vi "Complex Dot Product.vi"(2 "Y Vector":cdb[](array[numeric]) format="%.2f", 3 "X Vector":cdb[](array[numeric]) format="%.2f") -> (0 "error":i32, 1 "X * Y":cdb format="%.2f")   [LabVIEW 2017, in "NI_AALBase.lvlib"]
doc: "Computes the dot product of <B>X Vector</B> and <B>Y Vector</B>. The data types you wire to the <B>X Vector</B> and <B>Y Vector</B> inputs determine the polymorphic instance to use."
uses:
  NI_AALBase.lvlib
  <resource>/lvanlys.dll
panel:
  # "Complex Dot Product"
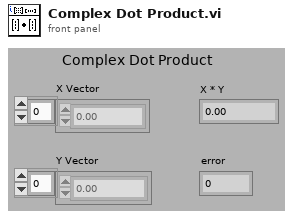
[diagram p1: front panel]
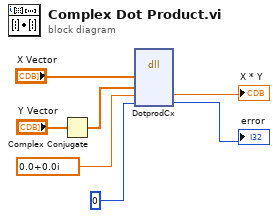
[diagram p0: block diagram]
diagram:
  n1 = Complex Conjugate(1:"Y Vector") -> (0:w1:cdb[])
  n2 = dll-call lib="C:/Program Files (x86)/National Instruments/LabVIEW 2017/resource/lvanlys.*" fn="DotprodCx"("X Vector"="X Vector", "output param"=w1, "output param"=cdb 0.0+0.0i, "output param"=0) -> ("output param"=→"X * Y":cdb, "output param"=→"error":i32)  [unwired: 6 in, 2 out]
